vi "setKey.vi"(7 "LegendProperties":T1={"Appearance"={"layout"="", "text-sample order"="", "key order"="", "surroundingBox"="", "MaxRows"=0, "MaxCols"=0, "WidthAdjust"=0.0}, "Alignment"={"Horizontal"="", "Vertical"=""}, "Location"="auto", "\"At\" location"={"XcoordSys"="", "YcoordSys"="", "Xvalue"=0.0, "Yvalue"=0.0}}, 8 "Set?":bool=TRUE, 11 "String in":string) -> (2 "command":string, 3 "String out":string)   [LabVIEW 2014]
uses:
  legendProperties.ctl
  legendAppearance.ctl
  alignment.ctl
  at.ctl
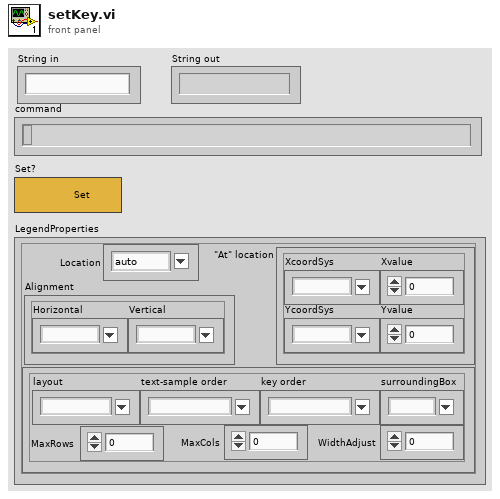
[diagram p1: front panel]
types:
  T1 = typedef "legendProperties.ctl" = cluster{"Appearance":T2, "Alignment":T3, "Location":string, "\"At\" location":T4}
  T2 = typedef "legendAppearance.ctl" = cluster{"layout":string, "text-sample order":string, "key order":string, "surroundingBox":string, "MaxRows":u32, "MaxCols":u32, "WidthAdjust":dbl}
  T3 = typedef "alignment.ctl" = cluster{"Horizontal":string, "Vertical":string}
  T4 = typedef "at.ctl" = cluster{"XcoordSys":string, "YcoordSys":string, "Xvalue":dbl, "Yvalue":dbl}
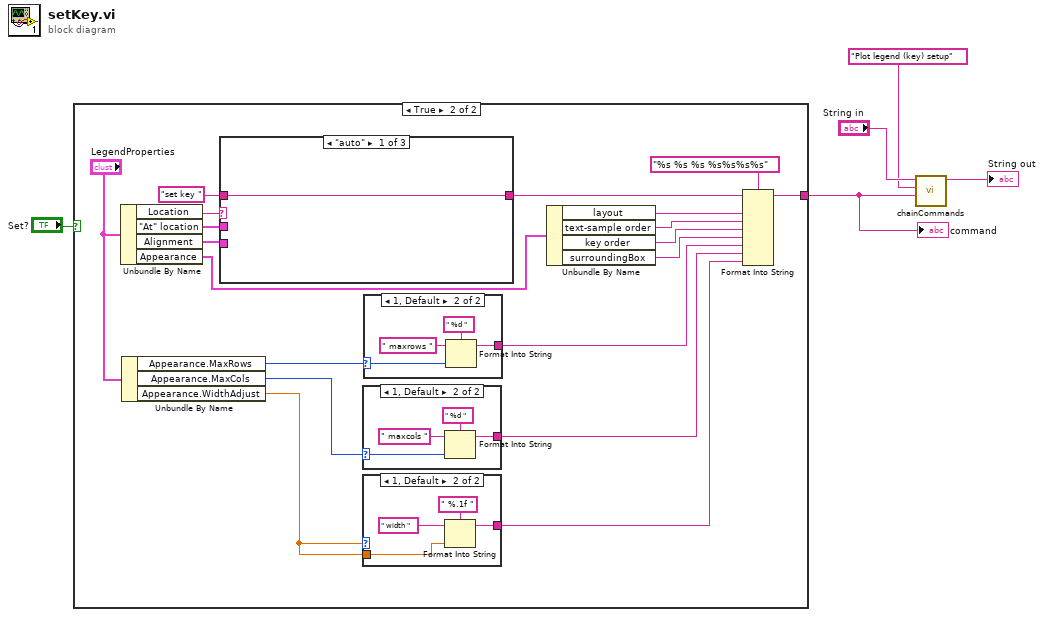
[diagram p0: block diagram]
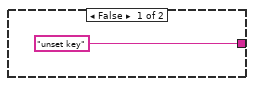
[diagram p2: hidden frame]
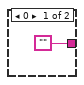
[diagram p3: hidden frame]
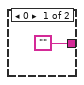
[diagram p4: hidden frame]
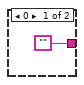
[diagram p5: hidden frame]
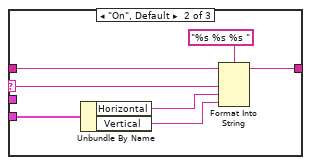
[diagram p6: hidden frame]
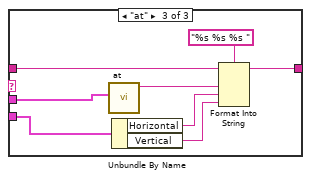
[diagram p7: hidden frame]
diagram:
  n1 = case shown="True" "Set?" {
    tunnel: ["unset key" w23] -> w3
    frame False {
    }
    frame True {
      n2 = Unbundle By Name("LegendProperties") -> ("Location"=w17:string, "\"At\" location"=w16:T4, "Alignment"=w15:T3, "Appearance"=w14:T2)
      n3 = Unbundle By Name("LegendProperties") -> ("Appearance.MaxRows"=w12:u32, "Appearance.MaxCols"=w10:u32, "Appearance.WidthAdjust"=w9:dbl)
      n4 = case shown="\"auto\"" w17 {
        selector: w17 -> [_ w42 _]
        tunnel: [w41 w48 w56] -> w22
        tunnel: "set key " -> [w41 w47 w55]
        tunnel: w15 -> [_ w43 w50]
        tunnel: w16 -> [_ _ w49]
        frame "auto" {
        }
        frame "On", Default {
          n5 = Unbundle By Name(w43) -> ("Horizontal"=w44:string, "Vertical"=w45:string)
          n6 = Format Into String(format string="%s %s %s ", initial string=w47, w42, w44, w45) -> (resulting string=w48:string)  [unwired: 1 in, 1 out]
        }
        frame "at" {
          n7 = call "at.vi"("\"At\" location"=w49) -> ("String out"=w53:string)  [unwired: 10 in]
          n8 = Unbundle By Name(w50) -> ("Horizontal"=w51:string, "Vertical"=w52:string)
          n9 = Format Into String(format string="%s %s %s ", initial string=w55, w53, w51, w52) -> (resulting string=w56:string)  [unwired: 1 in, 1 out]
        }
      }
      n10 = case shown="1, Default" w10 {
        selector: w10 -> [_ w32]
        tunnel: ["" w33] -> w8
        frame 0 {
        }
        frame 1, Default {
          n11 = Format Into String(format string=" %d ", initial string=" maxcols ", w32) -> (resulting string=w33:string)  [unwired: 1 in, 1 out]
        }
      }
      n12 = case shown="1, Default" w9 {
        tunnel: ["" w28] -> w7
        tunnel: w9 -> [_ w27]
        frame 0 {
        }
        frame 1, Default {
          n13 = Format Into String(format string=" %.1f ", initial string=" width ", w27) -> (resulting string=w28:string)  [unwired: 1 in, 1 out]
        }
      }
      n14 = case shown="1, Default" w12 {
        selector: w12 -> [_ w37]
        tunnel: ["" w38] -> w11
        frame 0 {
        }
        frame 1, Default {
          n15 = Format Into String(format string=" %d ", initial string=" maxrows ", w37) -> (resulting string=w38:string)  [unwired: 1 in, 1 out]
        }
      }
      n16 = Unbundle By Name(w14) -> ("layout"=w21:string, "text-sample order"=w20:string, "key order"=w19:string, "surroundingBox"=w18:string)
      n17 = Format Into String(format string="%s %s %s %s%s%s%s", initial string=w22, w21, w20, w19, w18, w11, w8, w7) -> (resulting string=w23:string)  [unwired: 1 in, 1 out]
    }
  }
  "command" <- w3
  n18 = call "chainCommands.vi"("Command"=w3, "Comments"="Plot legend (key) setup", "StringIn"="String in") -> ("StringOut"=→"String out":string)  [unwired: 8 in]
